vi "Adjust number of POI.vi"(6 "Ctrl refs":T1, 9 "Circles Data in":T2(array[cluster])) -> (1 "Circles Data out":T2(array[cluster]), 2 "Skipped":bool, 3 "Nb Circles out":i32)   [LabVIEW 2017]
uses:
  Typedefs/ROI entry screen ctrl refs cluster.ctl
  Typedefs/Line draw mode.ctl
  Typedefs/ROI move mode.ctl
  <userlib>/_OpenG.lib/numeric/numeric.llb/Random Number Within Range - I32__ogtk.vi
  <userlib>/_OpenG.lib/array/array.llb/Delete Elements from 1D Array (Variant)__ogtk.vi
panel:
  out "Multiplier (max = 1)":dbl
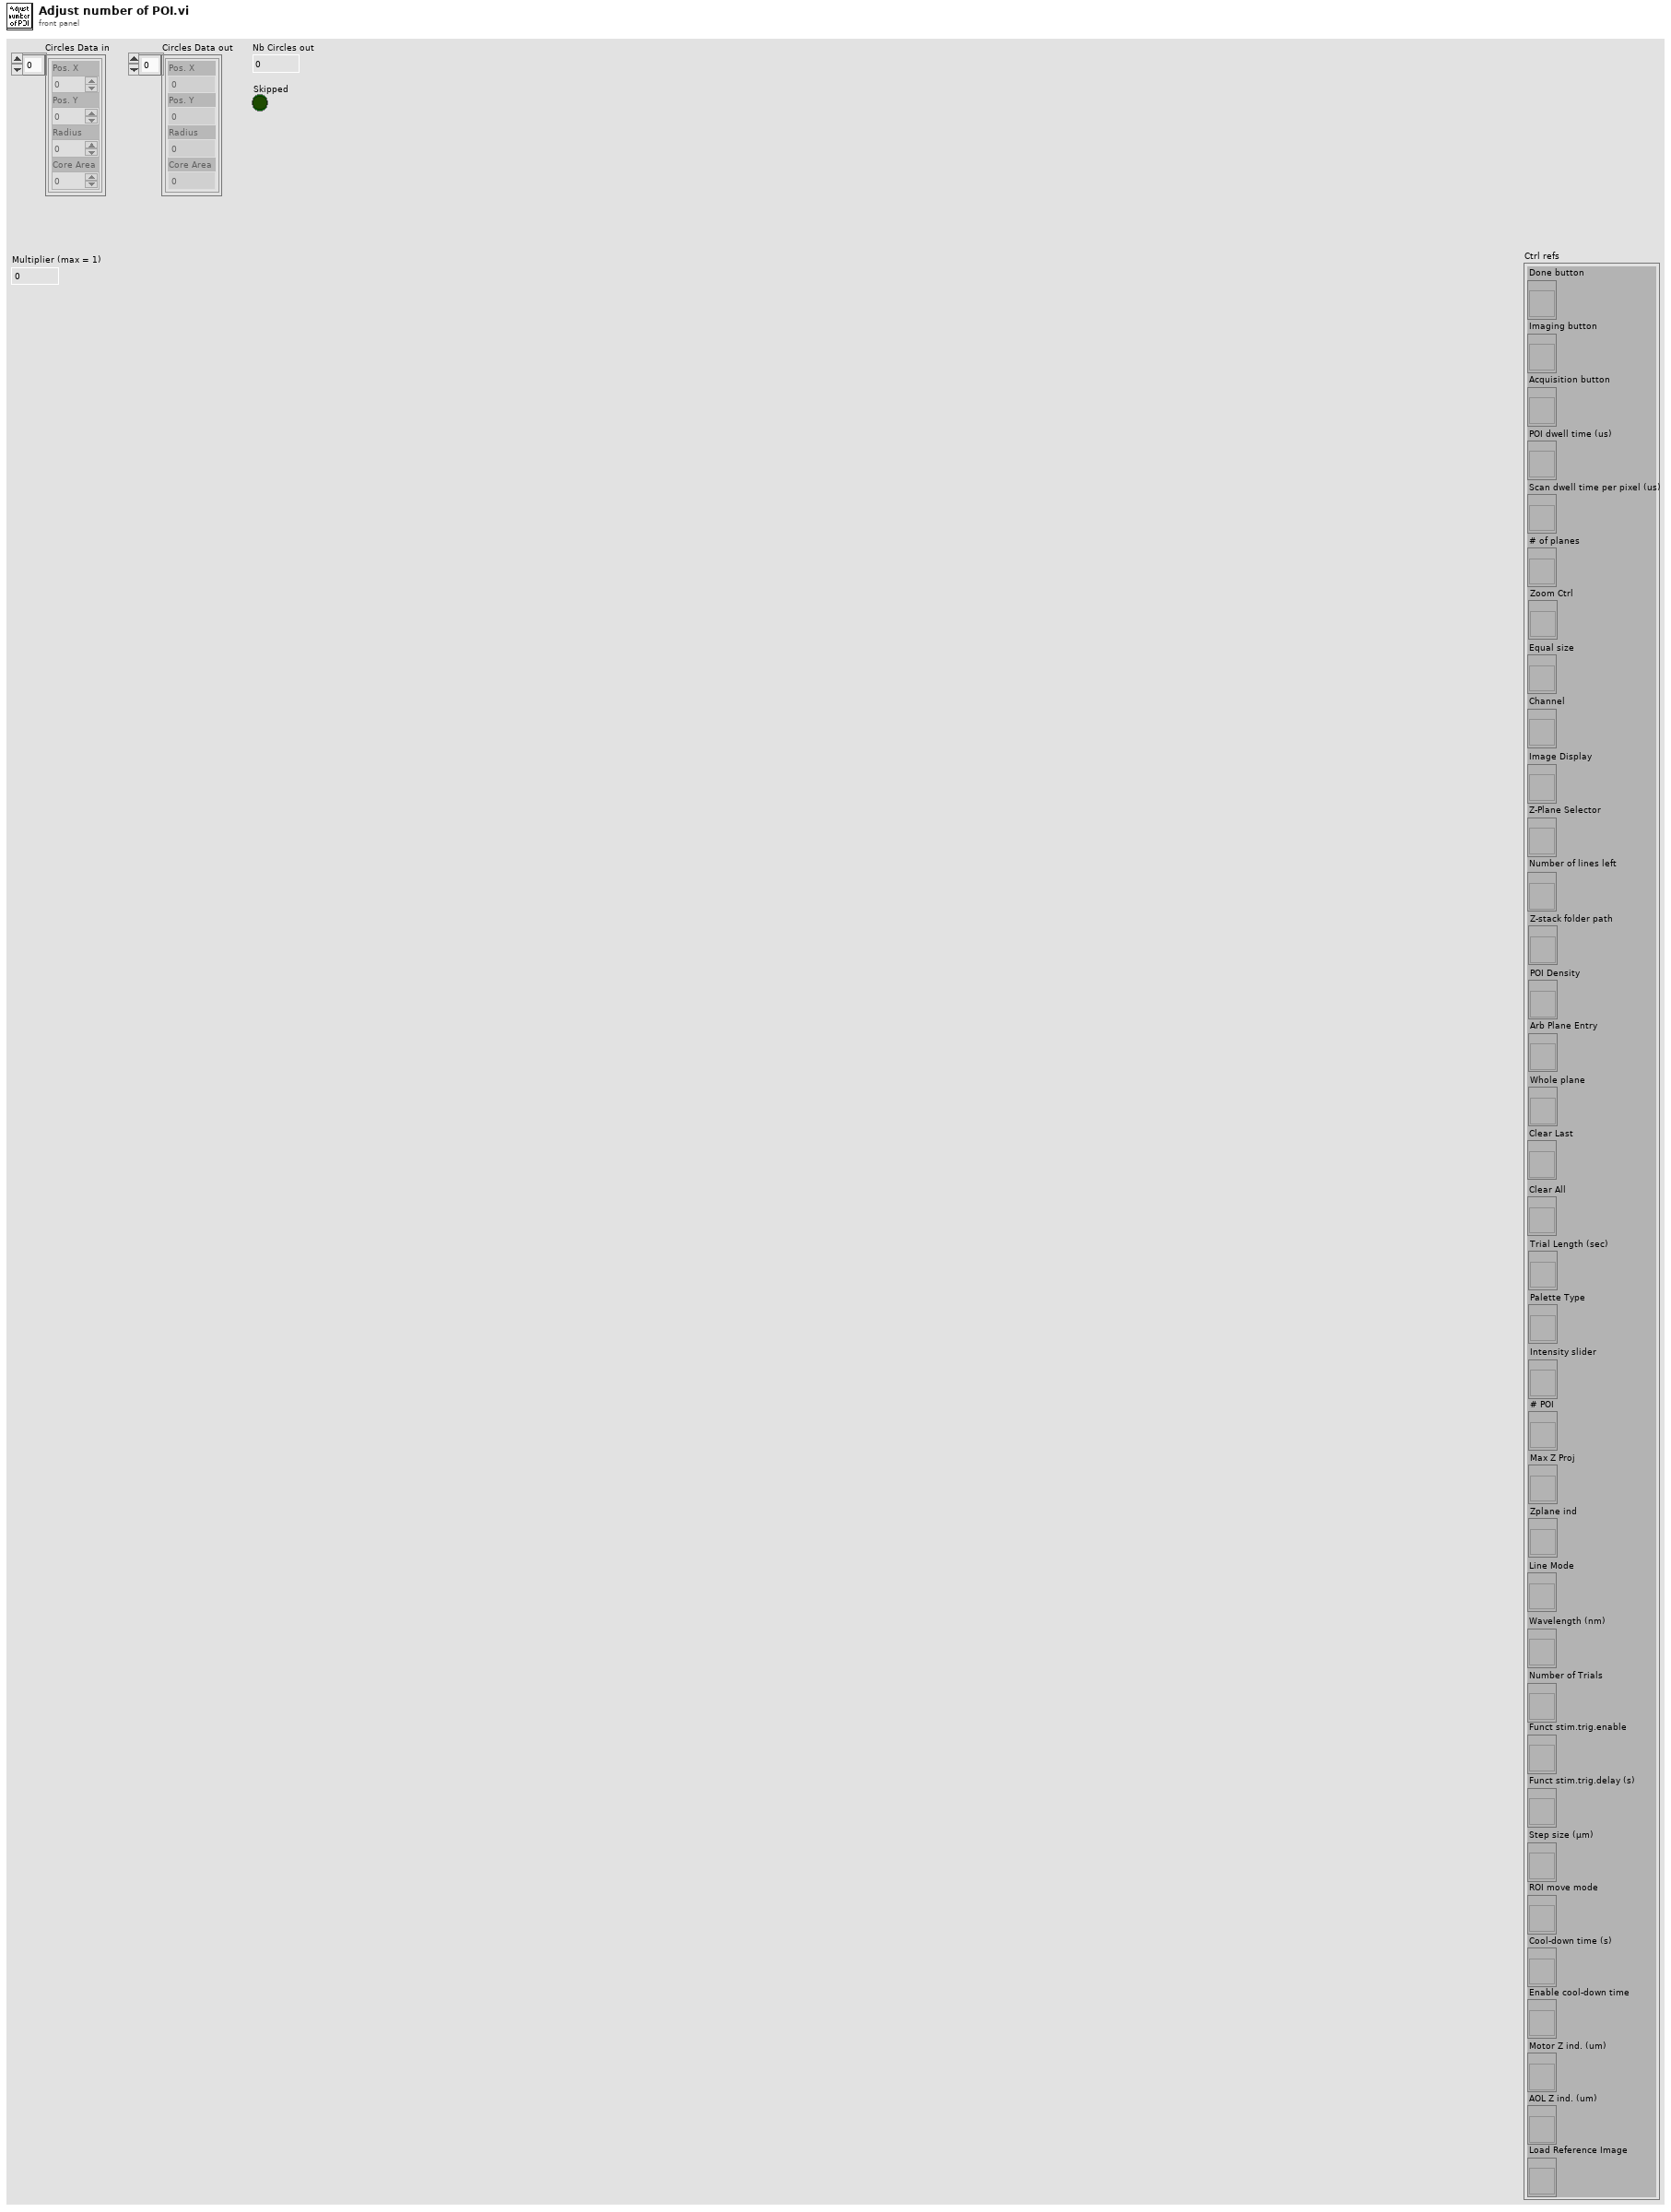
[diagram p1: front panel]
types:
  T1 = typedef "ROI entry screen ctrl refs cluster.ctl" = cluster{"Done button":refnum<vi>, "Imaging button":refnum<vi>, "Acquisition button":refnum<vi>, "POI dwell time (us)":refnum<vi>, "Scan dwell time per pixel (us)":refnum<vi>, "# of planes":refnum<vi>, "Zoom Ctrl":refnum<vi>, "Equal size":refnum<vi>, "Channel":refnum<vi>, "Image Display":refnum<vi>, "Z-Plane Selector":refnum<vi>, "Number of lines left":refnum<vi>, "Z-stack folder path":refnum<vi>, "POI Density":refnum<vi>, "Arb Plane Entry":refnum<vi>, "Whole plane":refnum<vi>, "Clear Last":refnum<vi>, "Clear All":refnum<vi>, "Trial Length (sec)":refnum<vi>, "Palette Type":refnum<vi>, "Intensity slider":refnum<vi>, "# POI":refnum<vi>, "Max Z Proj":refnum<vi>, "Zplane ind":refnum<vi>, "Wavelength (nm)":refnum<vi>, "Number of Trials":refnum<vi>, "Funct stim.trig.enable":refnum<vi>, "Funct stim.trig.delay (s)":refnum<vi>, "Line Mode":refnum<vi>, "Step size (µm)":refnum<vi>, "ROI move mode":refnum<vi>, "Cool-down time (s)":refnum<vi>, "Enable cool-down time":refnum<vi>, "Motor Z ind. (um)":refnum<vi>, "AOL Z ind. (um)":refnum<vi>, "Load Reference Image":refnum<vi>}
  T2 = cluster{"Pos. X":i32, "Pos. Y":i32, "Radius":i32, "Core Area":i32}[]
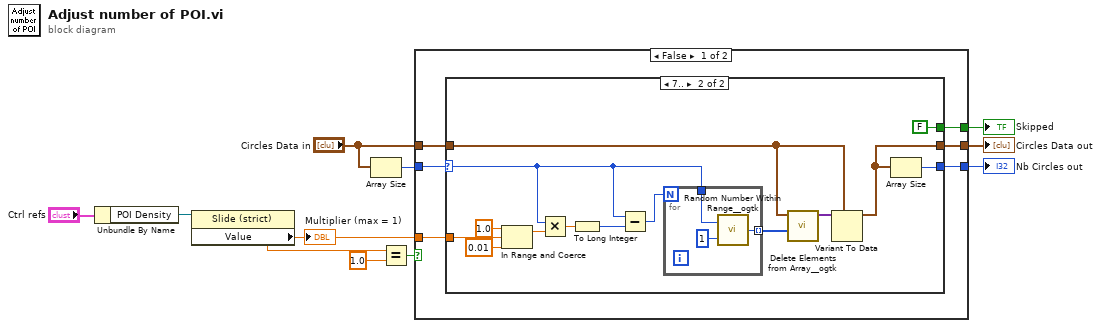
[diagram p0: block diagram]
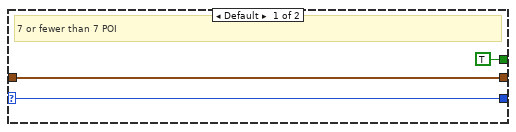
[diagram p2: hidden frame]
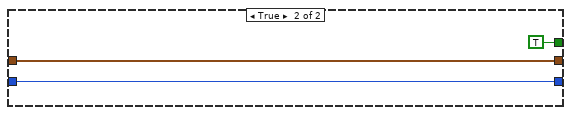
[diagram p3: hidden frame]
diagram:
  n1 = Unbundle By Name("Ctrl refs") -> ("POI Density"=w3:refnum<vi>)
  n2 = property class="Slide (strict)"(reference=w3) -> ("Value"=w1:dbl)  [unwired: 1 in, 2 out]
  "Multiplier (max = 1)" <- w1
  n3 = Array Size(array="Circles Data in") -> (size(s)=w4:i32)
  n4 = Equal?(x=w1, y=1.0) -> (x = y?=w7:bool)
  n5 = case shown="False" w7 {
    tunnel: w1 -> [w16 _]
    tunnel: "Circles Data in" -> [w14 w38]
    tunnel: [w13 w38] -> w10
    tunnel: w4 -> [w12 w37]
    tunnel: [w11 TRUE] -> w9
    tunnel: [w15 w37] -> w6
    frame False {
      n6 = case shown="7.." w12 {
        selector: w12 -> [w19 w21]
        tunnel: w14 -> [w18 w30]
        tunnel: [w18 w29] -> w13
        tunnel: [w19 w28] -> w15
        tunnel: w16 -> [_ w26]
        tunnel: [TRUE FALSE] -> w11
        frame Default {
          # "7 or fewer than 7 POI"
        }
        frame 7.. {
          n7 = In Range and Coerce(upper limit=1.0, x=w26, lower limit=0.01) -> (coerced(x)=w25:dbl)  [unwired: 1 out]
          n8 = Multiply(x=w21, y=w25) -> (x*y=w33:dbl)
          n9 = To Long Integer(number=w33) -> (32bit integer=w22:i32)
          n10 = Subtract(x=w21, y=w22) -> (x-y=w20:i32)
          n11 = for {
            N: w20 -> [_]
            tunnel: w21 -> [w36]
            tunnel: [w34] -> w32 mode=indexing
            n12 = call-poly <userlib>:"Random Number Within Range__ogtk.vi"("High"=w36, "Low"=1) -> ("Random Number"=w34:i32)  [unwired: 3 in]
          }
          n13 = call-poly <userlib>:"Delete Elements from Array__ogtk.vi"("indices"=w32, "array"=w30) -> ("array w/ subset deleted"=w31:variant[])  [unwired: 8 in, 1 out]
          n14 = Variant To Data(type=w30, Variant=w31) -> (data=w29:T2)  [unwired: 1 in, 1 out]
          n15 = Array Size(array=w29) -> (size(s)=w28:i32)
        }
      }
    }
    frame True {
    }
  }
  "Nb Circles out" <- w6
  "Circles Data out" <- w10
  "Skipped" <- w9
